vi "Analysator aktiv.vi"(6 "Aktion":T7, 8 "Autokal GT?":u16, 9 "Kalibrieren":T1, 10 "Aufschaltung CalGas":T2, 11 "Status Analysatoren":T6) -> (0 "Autokal GT?":u16, 1 "Kalibrieren":T1, 2 "Aufschaltung CalGas":T2, 3 "Status Analysatoren":T6)   [LabVIEW 2020, in "Allgemein.lvlib"]
uses:
  Allgemein.lvlib
  FGV Analysator aktiv.ctl
  Status Analysatoren/Status Analysatoren_Anzeige.ctl
  Seiten/CalGas Aufschaltung/Aufschaltung CalGas.ctl
  Visualisierungs Elemente/Auswahlfeld.ctl
  Seiten/CalGas Aufschaltung/Auswahl Aufschaltpunkt.ctl
  Seiten/CalGas Aufschaltung/Auswahl Analysator.ctl
  Auto Kalibrieren/KalibrierZustaende.ctl
  Status Analysatoren/Status Analysatoren.lvlib
  Seiten/CalGas Aufschaltung/CalGas Aufschaltung.lvlib
  Auto Kalibrieren/Auto Kalibrieren.lvlib
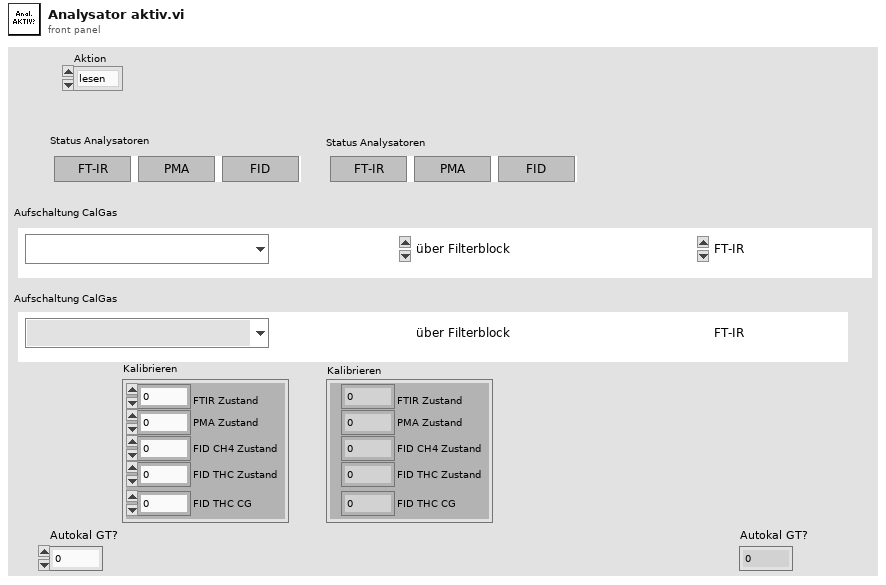
[diagram p1: front panel]
types:
  T1 = typedef "Auto Kalibrieren.lvlib/KalibrierZustaende.ctl" = cluster{"FTIR Zustand":u16, "PMA Zustand":u16, "FID CH4 Zustand":u16, "FID THC Zustand":u16, "FID THC CG":u16}
  T2 = typedef "CalGas Aufschaltung.lvlib/Aufschaltung CalGas.ctl" = cluster{"Kalibriergas":T3, "Aufschaltpunkt":T4, "Analysator":T5}
  T3 = typedef "Auswahlfeld.ctl" = u16
  T4 = typedef "CalGas Aufschaltung.lvlib/Auswahl Aufschaltpunkt.ctl" = enum16{"über Filterblock", "Analysator direkt", "über PNS", "Entnahme", "Gasdivider"}
  T5 = typedef "CalGas Aufschaltung.lvlib/Auswahl Analysator.ctl" = enum16{"FT-IR", "FID", "PMA", "PMA/FID/FT-IR"}
  T6 = typedef "Status Analysatoren.lvlib/Status Analysatoren_Anzeige.ctl" = cluster{"FT-IR":bool, "FID":bool, "PMA":bool}
  T7 = typedef "Allgemein.lvlib/FGV Analysator aktiv.ctl" = enum16{"lesen", "Analysator", "CG Aufschaltung", "KAL Zustand", "AutaKal GT?"}
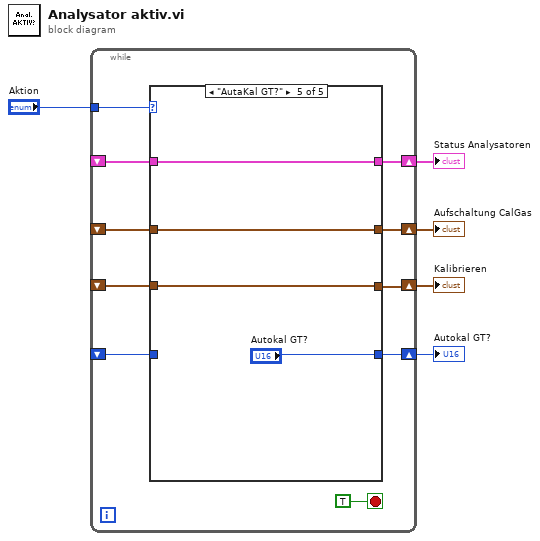
[diagram p0: block diagram]
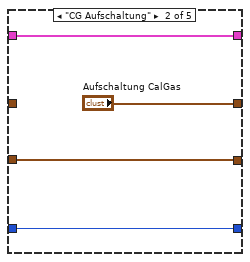
[diagram p3: hidden frame]
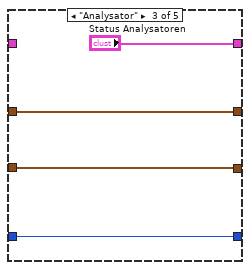
[diagram p4: hidden frame]
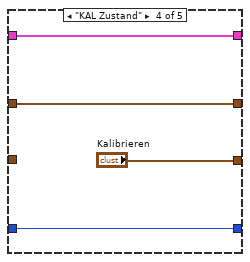
[diagram p5: hidden frame]
diagram:
  n1 = while {
    tunnel: "Aktion" -> [w14]
    shift-right: [w13] -> w4
    shift-left: _ -> [w12]
    shift-right: [w11] -> w3
    shift-left: _ -> [w10]
    shift-right: [w9] -> w2
    shift-left: _ -> [w8]
    shift-right: [w7] -> w1
    shift-left: _ -> [w6]
    stop <- TRUE stop-if-true
    n2 = case shown="\"AutaKal GT?\"" w14 {
      tunnel: [w19 w23 "Status Analysatoren" w29 w33] -> w13
      tunnel: w12 -> [w19 w23 _ w29 w33]
      tunnel: [w18 "Aufschaltung CalGas" w26 w30 w34] -> w11
      tunnel: w10 -> [w18 _ w26 w30 w34]
      tunnel: [w17 w21 w25 "Kalibrieren" w35] -> w9
      tunnel: w8 -> [w17 w21 w25 _ w35]
      tunnel: [w16 w20 w24 w28 "Autokal GT?"] -> w7
      tunnel: w6 -> [w16 w20 w24 w28 _]
      frame "lesen", Default {
      }
      frame "CG Aufschaltung" {
      }
      frame "Analysator" {
      }
      frame "KAL Zustand" {
      }
      frame "AutaKal GT?" {
      }
    }
  }
  "Status Analysatoren" <- w4
  "Aufschaltung CalGas" <- w3
  "Kalibrieren" <- w2
  "Autokal GT?" <- w1
